vi "ConnectVicon.vi"(11 "Mode":i32(ring) items=["ClientPull", "ClientPullPreFetch", "ServerPush"]) -> (0 "error out":errorcluster, 1 "Connected":bool, 3 ".NET Refnum out":refnum<k24>)   [LabVIEW 2024]
uses:
  C:/Users/ROAR/Documents/Rob Motor Assessment stuff/Labview/RobUST_3D_with_Unity_Control_PXI_Low_Level_Only_Streamlined/Vicon_files/ViconDataStreamSDK_DotNET.dll
  Vicon_files/ViconDataStreamSDK_DotNET.dll
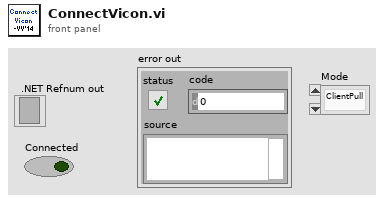
[diagram p1: front panel]
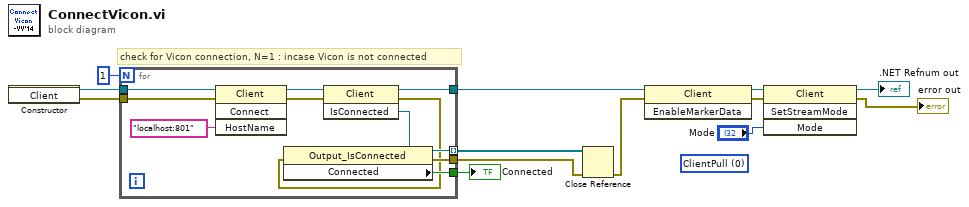
[diagram p0: block diagram]
diagram:
  (unwired) 0 items=["ClientPull", "ClientPullPreFetch", "ServerPush"] ("Mode")
  # "check for Vicon connection, N=1 : incase Vicon is not connected"
  n1 = constructor class="Client"() -> (reference out=w2:refnum<k24>, error out=w1:errorcluster)  [unwired: 3 in, 1 out]
  n2 = for {
    N: 1 -> [_]
    tunnel: w2 -> [w24]
    tunnel: [w21] -> w11
    tunnel: [w19] -> w13
    tunnel: w1 -> [w18]
    tunnel: [w16] -> w6 mode=indexing
    tunnel: [w15] -> w5
    n3 = invoke class="Client" method="Connect"(reference=w24, error in=w18, "HostName"="localhost:801") -> (reference out=w22:refnum<k24>, error out=w17:errorcluster)  [unwired: 1 in, 2 out]
    n4 = invoke class="Client" method="IsConnected"(reference=w22, error in=w17) -> (reference out=w21:refnum<k24>, error out=w14:errorcluster, "IsConnected"=w20:refnum<k24>)  [unwired: 1 in]
    n5 = property class="Output_IsConnected"(reference=w20, error in=w14) -> (reference out=w16:refnum<k24>, error out=w15:errorcluster, "Connected"=w19:bool)
  }
  "Connected" <- w13
  n6 = Close Reference(reference=w6, error in (no error)=w5) -> (error out=w4:errorcluster)
  n7 = invoke class="Client" method="EnableMarkerData"(reference=w11, error in=w4) -> (reference out=w10:refnum<k24>, error out=w8:errorcluster)  [unwired: 1 in, 1 out]
  n8 = invoke class="Client" method="SetStreamMode"(reference=w10, error in=w8, "Mode"="Mode") -> (reference out=→".NET Refnum out":refnum<k24>, error out=→"error out":errorcluster)  [unwired: 1 in, 2 out]
